vi "Initialize Engine.vi"(8 "error in":errorcluster, 10 "settings in":T2, 11 "Device Reference in":T8 format="%.0x") -> (0 "error out":errorcluster, 1 "inline runtime data":T1, 2 "settings out":T2, 3 "Device Reference out":T8 format="%.0x")   [LabVIEW 2019, in "HLA Custom Device Engine.lvlib"]
uses:
  HLA Custom Device Engine.lvlib
  <vilib>/NI VeriStand/Custom Device API/Custom Device Item Ref.ctl
  Shared/Compiled.Settings.ctl
  Shared/main_page_config.ctl
  Shared/object_managament_config.ctl
  Shared/interaction_parameter_configuration.ctl
  Shared/object_attribute_configuration.ctl
  Shared/object_status_info.ctl
  RTinlineRuntimeData.ctl
  _Debug/VsDebugLibrary.lvlib
  <vilib>/NI VeriStand/Custom Device API/Custom Device API.lvlib
  Shared/HLA Custom Device Shared.lvlib
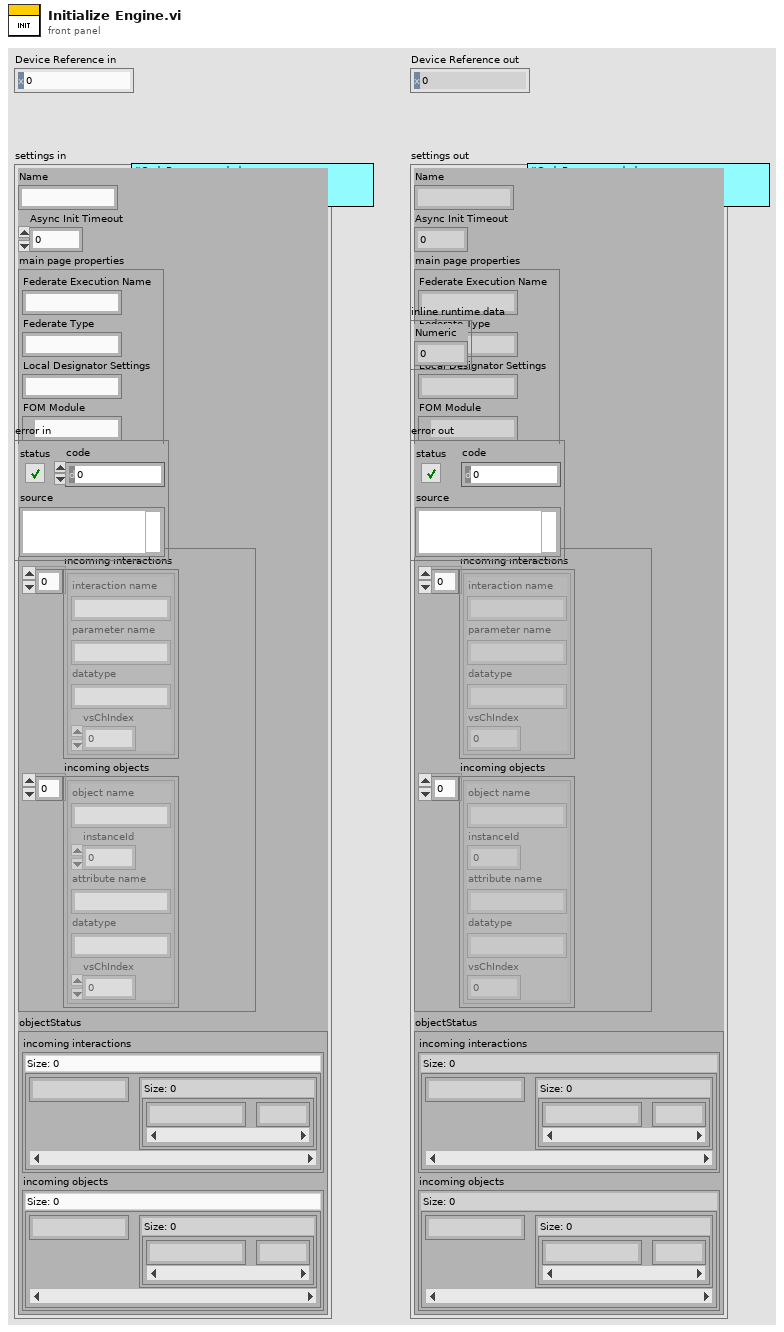
[diagram p1: front panel]
types:
  T1 = typedef "HLA Custom Device Engine.lvlib/RTinlineRuntimeData.ctl" = cluster{"Numeric":dbl}
  T2 = typedef "HLA Custom Device Shared.lvlib/Compiled.Settings.ctl" = cluster{"Name":string, "Async Init Timeout":u16, "main page properties":T3, "obiectConfig":T4, "objectStatus":T7}
  T3 = typedef "HLA Custom Device Shared.lvlib/main_page_config.ctl" = cluster{"Federate Execution Name":string, "Federate Type":string, "Local Designator Settings":string, "FOM Module":path, "mak mtl file":path, "FOM destination path":string}
  T4 = typedef "HLA Custom Device Shared.lvlib/object_managament_config.ctl" = cluster{"incoming interactions":T5[], "incoming objects":T6[]}
  T5 = typedef "HLA Custom Device Shared.lvlib/interaction_parameter_configuration.ctl" = cluster{"interaction name":string, "parameter name":string, "datatype":string, "vsChIndex":i32}
  T6 = typedef "HLA Custom Device Shared.lvlib/object_attribute_configuration.ctl" = cluster{"object name":string, "instanceId":i32, "attribute name":string, "datatype":string, "vsChIndex":i32}
  T7 = typedef "HLA Custom Device Shared.lvlib/object_status_info.ctl" = cluster{"incoming interactions":map{string, map{string, i32}}, "incoming objects":map{string, map{string, i32}}}
  T8 = typedef "Custom Device API.lvlib/Custom Device Item Ref.ctl" = u64
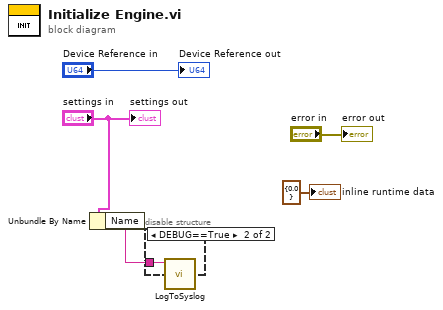
[diagram p0: block diagram]
diagram:
  n1 = Unbundle By Name("settings in") -> ("Name"=w1:string)
  n2 = disable-structure shown="DEBUG==True" {
    disable-tunnel: w1 -> [_ w6]
    frame condition #0 {
    }
    frame condition #1 (active) {
      n3 = call "LogToSyslog.vi"("message"=w6) -> ()  [unwired: 9 in, 2 out]
    }
  }
  "Device Reference out" <- "Device Reference in"
  "settings out" <- "settings in"
  "error out" <- "error in"
  "inline runtime data" <- T1 {"Numeric"=0.0} ("inline runtime data")
